vi "I2C_TRANSFER_n.vi"(2 "execute":bool, 7 "uLPtr":u32[](array[numeric]), 11 "error in (no error)":errorcluster) -> (4 "function return":string, 6 "ulValue":u32, 8 "uLPtr":u32[](array[numeric]), 10 "BytePtr":u8[](array[numeric]), 15 "error out":errorcluster)   [LabVIEW 2017, in "ZBOX_IS.lvlib"]
uses:
  ZBOX_IS.lvlib
panel:
  out "Numeric":i32
  out "x > 0?":bool
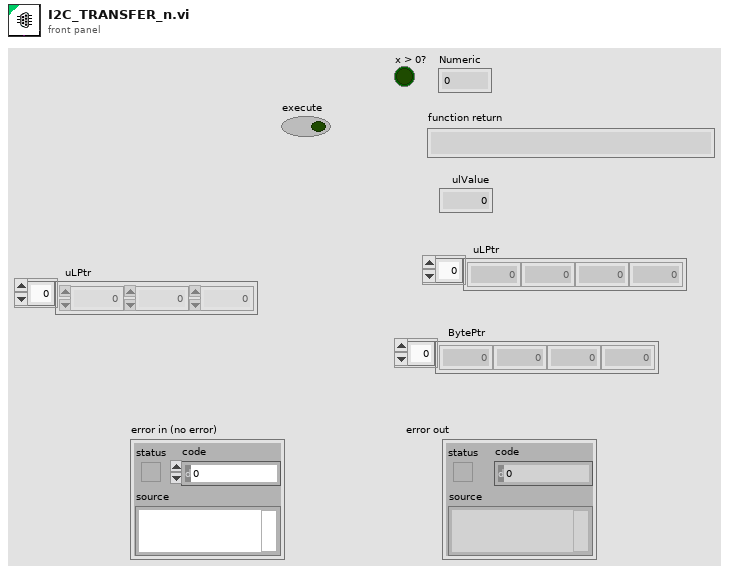
[diagram p1: front panel]
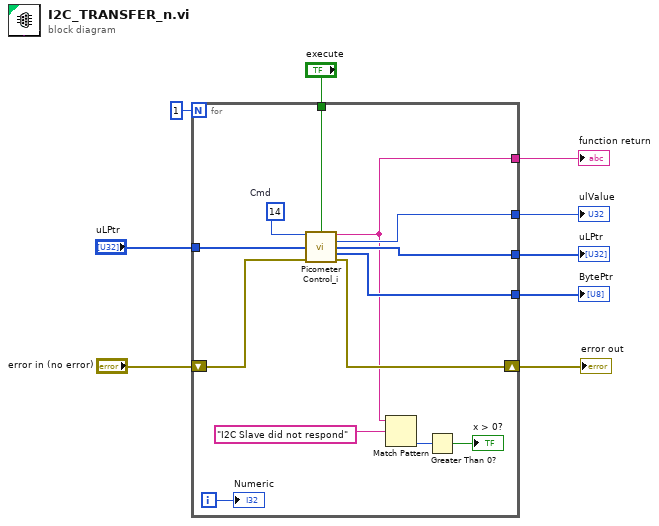
[diagram p0: block diagram]
diagram:
  n1 = for {
    N: 1 -> [_]
    tunnel: [w14] -> w7
    tunnel: [w18] -> w5
    tunnel: [w17] -> w4
    tunnel: "execute" -> [w15]
    shift-right: [w20] -> w8
    shift-left: "error in (no error)" -> [w21]
    tunnel: "uLPtr" -> [w16]
    tunnel: [w19] -> w6
    i -> [w11]
    w22 = u8 14  # Cmd
    n2 = call "Picometer Control_i.vi"("Cmd"=w22, "execute"=w15, "uLPtr"=w16, "error in (no error)"=w21) -> ("function return"=w14:string, "ulValue"=w17:u32, "uLPtr"=w19:u32[], "BytePtr"=w18:u8[], "error out"=w20:errorcluster)  [unwired: 7 in]
    n3 = Match Pattern(string=w14, regular expression="I2C Slave did not respond" ("function return 2")) -> (offset past match=w12:i32)  [unwired: 1 in, 3 out]
    n4 = Greater Than 0?(x=w12) -> (x > 0?=→"x > 0?":bool)
    "Numeric" <- w11
  }
  "error out" <- w8
  "function return" <- w7
  "uLPtr" <- w6
  "BytePtr" <- w5
  "ulValue" <- w4
